vi "File.Search Folder for Files baed on Pattern, Sort based on Modified Data.vi"(8 "error in":errorcluster, 9 "Sort (T = New to Old)":bool=TRUE, 10 "Pattern":string, 11 "Folder":path) -> (0 "error out":errorcluster, 3 "Matched Files":path[](array[path]))   [LabVIEW 2019]
panel:
  out "Files":cluster{"last mod":timestamp, "path out":path}[](array[cluster])
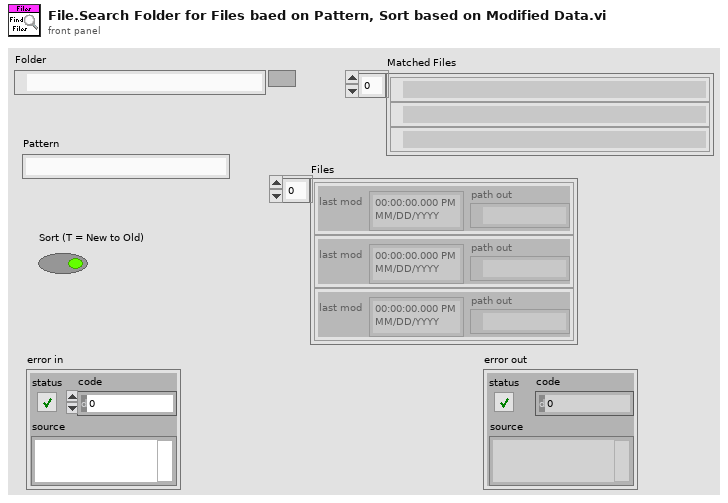
[diagram p1: front panel]
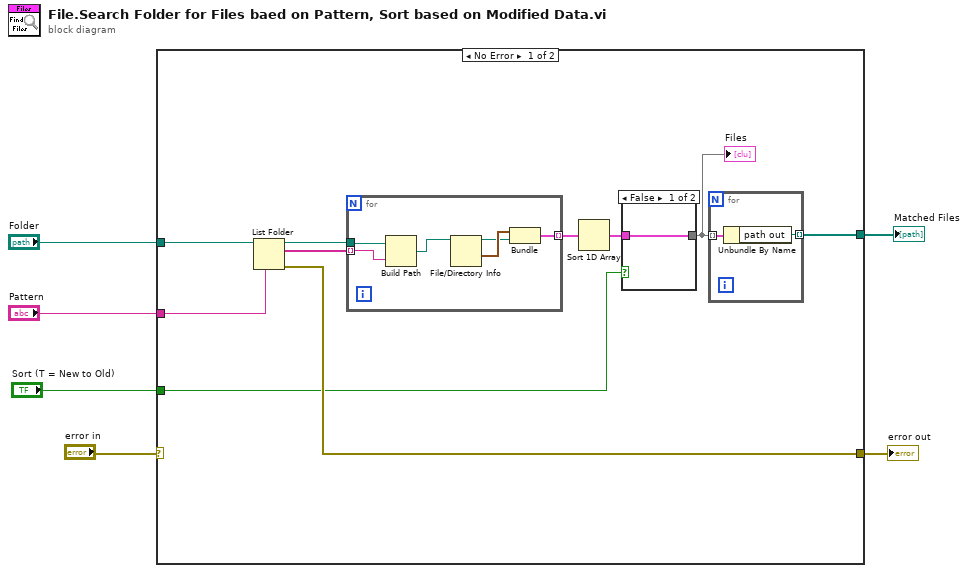
[diagram p0: block diagram]
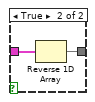
[diagram p2: hidden frame]
diagram:
  n1 = case shown="No Error" "error in" {
    selector: "error in" -> [_ w28]
    tunnel: "Folder" -> [w16 _]
    tunnel: "Pattern" -> [w15 _]
    tunnel: [w14 w28] -> w3
    tunnel: [w8 _] -> w2
    tunnel: "Sort (T = New to Old)" -> [w7 _]
    frame No Error {
      n2 = List Folder(path=w16, pattern=w15) -> (path out=w12:path, filenames=w13:string[], error out=w14:errorcluster)  [unwired: 2 in, 1 out]
      n3 = for {
        tunnel: w13 -> [w26] mode=indexing
        tunnel: w12 -> [w27]
        tunnel: [w22] -> w11 mode=indexing
        n4 = Build Path(base path=w27, name or relative path=w26) -> (appended path=w25:path)
        n5 = File/Directory Info(path=w25) -> (path out=w23:path, last mod=w24:timestamp)  [unwired: 1 in, 5 out]
        n6 = Bundle("last mod"=w24, "path out"=w23) -> (w22:cluster{"last mod":timestamp, "path out":path})  [unwired: 1 in]
      }
      n7 = Sort 1D Array(array=w11) -> (sorted array=w10:cluster{"last mod":timestamp, "path out":path}[])
      n8 = case shown="False" w7 {
        tunnel: w10 -> [w17 w19]
        tunnel: [w17 w18] -> w9
        frame False {
        }
        frame True {
          n9 = Reverse 1D Array(array=w19) -> (reversed array=w18:cluster{"last mod":timestamp, "path out":path}[])
        }
      }
      "Files" <- w9
      n10 = for {
        tunnel: w9 -> [w21] mode=indexing
        tunnel: [w20] -> w8 mode=indexing
        n11 = Unbundle By Name(w21) -> ("path out"=w20:path)
      }
    }
    frame Error {
    }
  }
  "Matched Files" <- w2
  "error out" <- w3
